vi "DisconnectDevice.vi"(8 "Error in":errorcluster, 11 "DevicesAndSignals":T1) -> (0 "Error out":errorcluster)   [LabVIEW 2016]
doc: "Disconnects all given devices.\n\nDevices: Array of devices to disconnect"
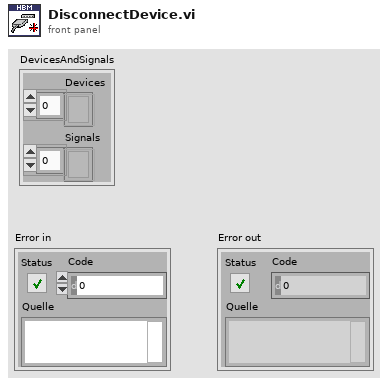
[diagram p1: front panel]
types:
  T1 = cluster{"Devices":refnum<k24>[], "Signals":refnum<k24>[]}
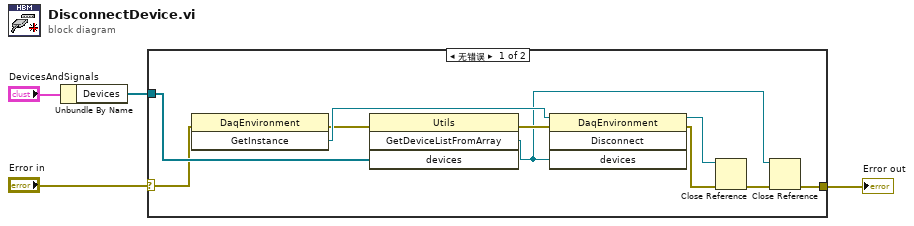
[diagram p0: block diagram]
diagram:
  n1 = Unbundle By Name("DevicesAndSignals") -> ("Devices"=w1:refnum<k24>[])
  n2 = case shown="无错误" "Error in" {
    selector: "Error in" -> [w12 w15]
    tunnel: [w5 w15] -> w3
    tunnel: w1 -> [w13 _]
    frame No Error {
      n3 = invoke on="Methodenknoten" class="DaqEnvironment" method="GetInstance"(error in=w12) -> (error out=w10:errorcluster, "GetInstance"=w11:refnum<k24>)  [unwired: 2 in, 1 out]
      n4 = invoke on="Methodenknoten" class="Utils" method="GetDeviceListFromArray"(error in=w10, "devices"=w13) -> (error out=w14:errorcluster, "GetDeviceListFromArray"=w6:refnum<k24>)  [unwired: 2 in, 2 out]
      n5 = invoke class="DaqEnvironment" method="Disconnect"(reference=w11, error in=w14, "devices"=w6) -> (reference out=w8:refnum<k24>, error out=w9:errorcluster)  [unwired: 1 in, 2 out]
      n6 = Close Reference(reference=w8, error in (no error)=w9) -> (error out=w7:errorcluster)
      n7 = Close Reference(reference=w6, error in (no error)=w7) -> (error out=w5:errorcluster)
    }
    frame Error {
    }
  }
  "Error out" <- w3
